vi "编码器角度位置测量_有限.vi"() -> ()   [LabVIEW 2013]
uses:
  <userlib>/ArtDAQ/_SubVI/ArtDAQ_CreateCIAngEncoderChan.vi
  <userlib>/ArtDAQ/_SubVI/ArtDAQ_CfgSampClkTiming.vi
  <userlib>/ArtDAQ/_SubVI/ArtDAQ_Read Counter DBL NSamp.vi
panel:
  in  "Z索引相位":i32(ring)=10040 items=["A高B高"=10040, "A高B低"=10041, "A低B高"=10042, "A低B低"=10043]
  in  "解码类型":i32(ring)=10090 items=["X1"=10090, "X2"=10091, "X4"=10092, "TwoPulse"=10313]
  in  "时钟源":string="/Dev1/PFI0"
  in  "初始角度":dbl
  in  "脉冲/转":u32=24
  in  "Z索引值":dbl
  in  "启用Z索引":bool
  in  "每通道点数":i32=100
  out "数据":dbl[](array[numeric])
  in  "计数器":string="Dev1/ctr0"
  in  "采样频率":dbl=1000.0 caption="采样速率" format="%0.6f"
  out "错误输出":errorcluster
  # "通道属性"
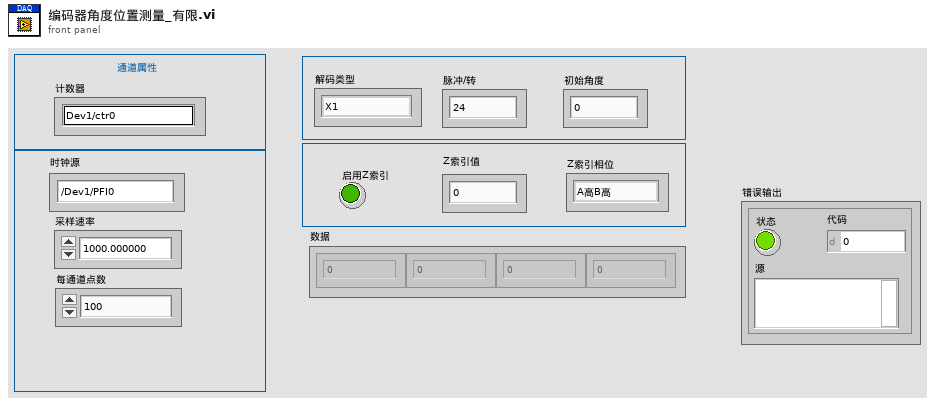
[diagram p1: front panel]
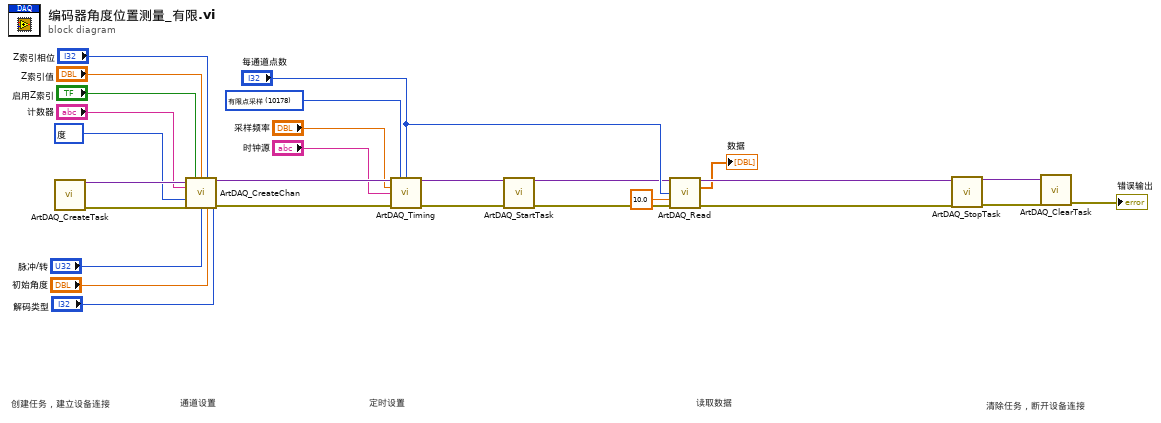
[diagram p0: block diagram]
diagram:
  w10 = 10146 items=["度"=10146, "弧度"=10273, "时钟滴答"=10304, "来自自定义换算"=10065] ("单位")
  w15 = 10178 items=["有限点采样"=10178, "连续采样"=10123] ("SampleMode")
  # "清除任务，断开设备连接"
  # "读取数据"
  # "定时设置"
  # "通道设置"
  # "创建任务，建立设备连接"
  n1 = call <userlib>:"ArtDAQ_CreateTask.vi"() -> ("任务句柄"=w27:variant, "错误输出"=w26:errorcluster)  [unwired: 14 in]
  n2 = call-poly <userlib>:"ArtDAQ_CreateChan.vi"("任务句柄"=w27, "启用Z索引"="启用Z索引", "Z索引值"="Z索引值", "Z索引相位"="Z索引相位", "计数器"="计数器", "解码类型"="解码类型", "单位"=w10, "错误输入"=w26, "脉冲每转"="脉冲/转", "初始角"="初始角度") -> ("任务句柄"=w19:variant, "错误输出"=w17:errorcluster)  [unwired: 4 in]
  n3 = call-poly <userlib>:"ArtDAQ_Timing.vi"("任务句柄"=w19, "采样模式"=w15, "每通道采样数"="每通道点数", "采样率"="采样频率", "源"="时钟源", "错误输入"=w17) -> ("任务句柄"=w18:variant, "错误输出"=w16:errorcluster)  [unwired: 8 in]
  n4 = call <userlib>:"ArtDAQ_StartTask.vi"("任务句柄"=w18, "错误输入"=w16) -> ("任务句柄"=w7:variant, "错误输出"=w6:errorcluster)  [unwired: 12 in]
  n5 = call-poly <userlib>:"ArtDAQ_Read.vi"("任务句柄"=w7, "每通道采样数"="每通道点数", "超时s"=10.0 ("Timeout"), "错误输入"=w6) -> ("任务句柄"=w24:variant, "数据"=→"数据":dbl[], "错误输出"=w22:errorcluster)  [unwired: 8 in, 1 out]
  n6 = call <userlib>:"ArtDAQ_StopTask.vi"("任务句柄"=w24, "错误输入"=w22) -> ("任务句柄"=w23:variant, "错误输出"=w21:errorcluster)  [unwired: 12 in]
  n7 = call <userlib>:"ArtDAQ_ClearTask.vi"("任务句柄"=w23, "错误输入"=w21) -> ("错误输出"=→"错误输出":errorcluster)  [unwired: 13 in]
